vi "Get Connections - 1Pin MConn.vi"(6 "pin type":T3, 8 "error in":errorcluster, 9 "site":i32, 10 "pin or relay name":string, 11 "session reservation in":refnum<class "Session Reservation.lvclass">) -> (0 "error out":errorcluster, 2 "connections":T1[](array[typedef]), 3 "session reservation out":refnum<class "Session Reservation.lvclass">)   [LabVIEW 2021, in "Session Management niDAQmx.lvlib"]
uses:
  Session Management niDAQmx.lvlib
  <vilib>/Plug-In SDKs/Clients/Session Management V1/Session Reservation/Pin Type.ctl
  <vilib>/Plug-In SDKs/Clients/Session Management V1/Session Reservation/Session Reservation.lvclass
  Connection with Session.ctl
  Session Factory/Session Factory.lvclass
  C:/Program Files/National Instruments/LabVIEW 2021/vi.lib/Plug-In SDKs/Sessions/Instrument/ISession Factory/ISession Factory.lvclass
  <vilib>/Plug-In SDKs/Clients/Session Management V1/Session Reservation/Connection.ctl
  79dae63b-3509-4808-af52-6d4f0ce28fba.vi
  79dae63b-3509-4808-af52-6d4f0ce28fba.vi/10aac40e-32b1-41e4-9263-c4508fa95940.vi
  <vilib>/Plug-In SDKs/Clients/Session Management V1/Session Reservation/Pin to Pin Array.vi
  <vilib>/Plug-In SDKs/Clients/Session Management V1/Session Reservation/Get Connections Impl.vi
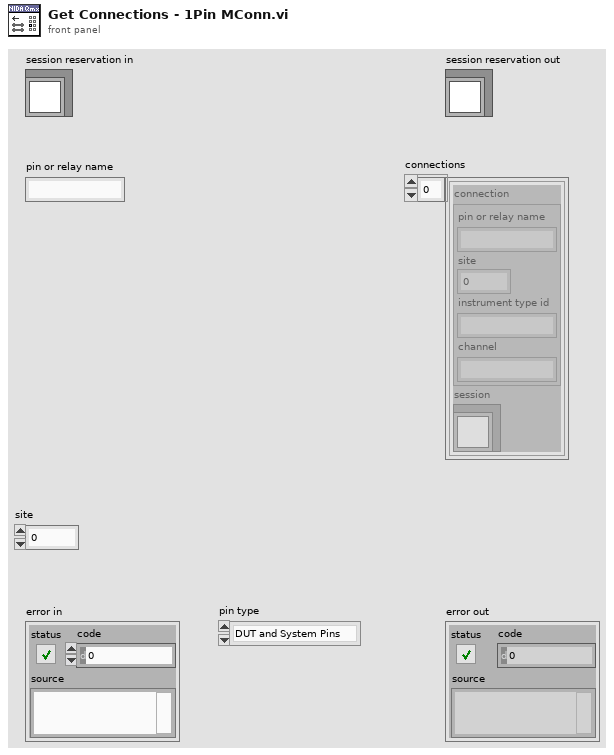
[diagram p1: front panel]
types:
  T1 = typedef "Session Management niDAQmx.lvlib/Connection with Session.ctl" = cluster{"connection":T2, "session":refnum<class "Session Factory.lvclass">}
  T2 = typedef "NI Session Management V1 Client.lvlib/Session Reservation.lvclass/Connection.ctl" = cluster{"pin or relay name":string, "site":i32, "instrument type id":string, "channel":string}
  T3 = typedef "NI Session Management V1 Client.lvlib/Session Reservation.lvclass/Pin Type.ctl" = enum16{"DUT and System Pins", "System Pins"}
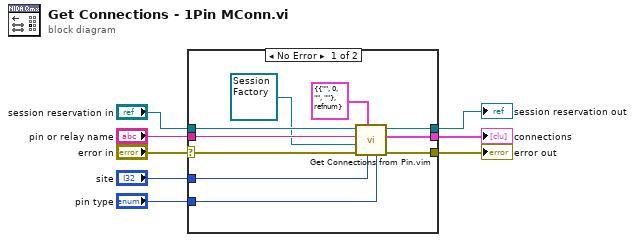
[diagram p0: block diagram]
diagram:
  n1 = case shown="No Error" "error in" {
    selector: "error in" -> [w18 w20]
    tunnel: "site" -> [w10 _]
    tunnel: "pin type" -> [w9 _]
    tunnel: [w17 w20] -> w5
    tunnel: "pin or relay name" -> [w13 _]
    tunnel: "session reservation in" -> [w14 w19]
    tunnel: [w15 w19] -> w2
    tunnel: [w16 _] -> w1
    frame No Error {
      n2 = call "Get Connections from Pin.vim"("pin type"=w9, "site"=w10, "connection type"=T1 {"connection"={"pin or relay name"="", "site"=0, "instrument type id"="", "channel"=""}, "session"=refnum} ("connection with task"), "error in"=w18, "session factory"=refnum<class "Session Factory.lvclass"> refnum ("Session Management niDAQmx.lvlib:Session Factory.lvclass"), "pin or relay name"=w13, "session reservation in"=w14) -> ("error out"=w17:errorcluster, "connections"=w16:T1[], "session reservation out"=w15:refnum<class "Session Reservation.lvclass">)  [unwired: 2 in]
    }
    frame Error {
    }
  }
  "error out" <- w5
  "session reservation out" <- w2
  "connections" <- w1
